vi "TpTcpError.vi"() -> (1 "tracepoint name":string)   [LabVIEW 2017, in "ServerComm.lvlib"]
uses:
  <vilib>/addons/InsightCM/Devices/Shared/Common/ServerComm/ServerComm.lvlib
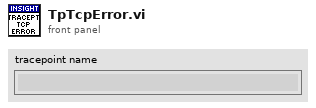
[diagram p1: front panel]
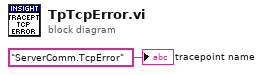
[diagram p0: block diagram]
diagram:
  "tracepoint name" <- "ServerComm.TcpError" ("ProcessName")
